vi "ControlsToCommands.vi"(11 "input cluster":T1) -> (3 "output cluster":T2)   [LabVIEW 2015]
uses:
  ControlsToCommands.ctl
  Controls.ctl
  Robot Global Data.vi
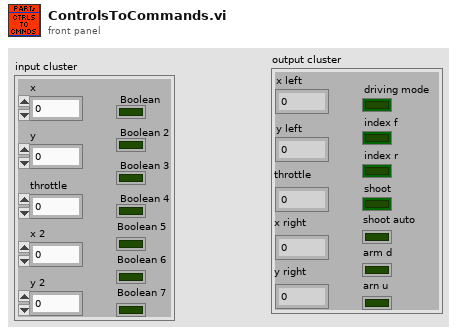
[diagram p1: front panel]
types:
  T1 = typedef "Controls.ctl" = cluster{"x":dbl, "y":dbl, "throttle":dbl, "x 2":dbl, "y 2":dbl, "Boolean":bool, "Boolean 2":bool, "Boolean 3":bool, "Boolean 4":bool, "Boolean 5":bool, "Boolean 6":bool, "Boolean 7":bool}
  T2 = typedef "ControlsToCommands.ctl" = cluster{"x left":dbl, "y left":dbl, "throttle":dbl, "x right":dbl, "y right":dbl, "driving mode":bool, "index f":bool, "index r":bool, "shoot":bool, "shoot auto":bool, "arm d":bool, "arn u":bool}
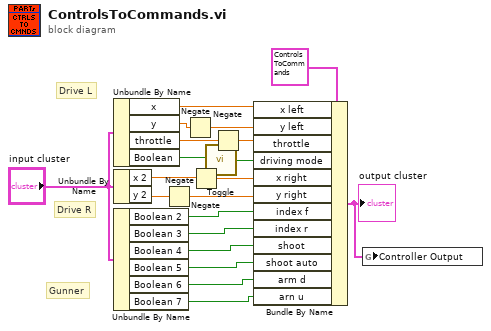
[diagram p0: block diagram]
diagram:
  # "Gunner"
  # "Drive R"
  # "Drive L"
  n1 = Unbundle By Name("input cluster") -> ("x"=w1:dbl, "y"=w10:dbl, "throttle"=w7:dbl, "Boolean"=w11:bool)
  n2 = Unbundle By Name("input cluster") -> ("x 2"=w3:dbl, "y 2"=w5:dbl)
  n3 = Unbundle By Name("input cluster") -> ("Boolean 2"=w18:bool, "Boolean 3"=w17:bool, "Boolean 4"=w16:bool, "Boolean 5"=w15:bool, "Boolean 6"=w14:bool, "Boolean 7"=w13:bool)
  n4 = Negate(x=w5) -> (-x=w6:dbl)
  n5 = Negate(x=w10) -> (-x=w9:dbl)
  n6 = Negate(x=w3) -> (-x=w4:dbl)
  n7 = call "Toggle.vi"("Input"=w11) -> ("Output"=w12:bool)  [unwired: 4 in]
  n8 = Negate(x=w7) -> (-x=w8:dbl)
  n9 = Bundle By Name(cluster=T2 {"x left"=0.0, "y left"=0.0, "throttle"=0.0, "x right"=0.0, "y right"=0.0, "driving mode"=FALSE, "index f"=FALSE, "index r"=FALSE, "shoot"=FALSE, "shoot auto"=FALSE, "arm d"=FALSE, "arn u"=FALSE} ("input cluster"), "x left"=w1, "y left"=w9, "throttle"=w8, "driving mode"=w12, "x right"=w4, "y right"=w6, "index f"=w18, "index r"=w17, "shoot"=w16, "shoot auto"=w15, "arm d"=w14, "arn u"=w13) -> (w2:T2)
  "output cluster" <- w2
  n10 = global write "Robot Global Data.vi" "Controller Output"(w2) -> ()
